vi "Block touchscreen.vi"(8 "error in (no error)":errorcluster, 10 "Block touchscreen?":bool, 11 "VISA resource name":refnum<visa-resource-name>) -> (0 "error out":errorcluster, 3 "VISA resource name out":refnum<visa-resource-name>)   [LabVIEW 2017, in "Sefram DAS220.lvlib"]
doc: "Lock or unlock the device touchscreen."
uses:
  <instrlib>/Sefram DAS220/Sefram DAS220.lvlib
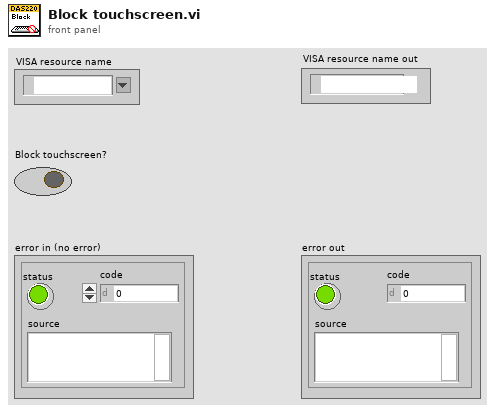
[diagram p1: front panel]
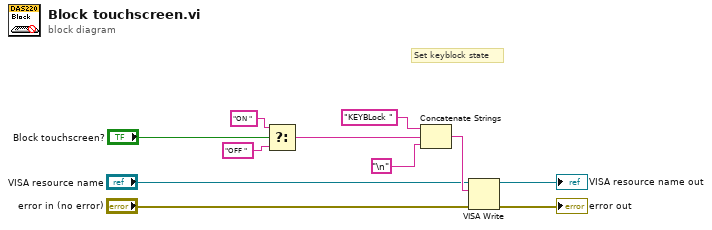
[diagram p0: block diagram]
diagram:
  # "Set keyblock state"
  n1 = Select(t="ON " ("string"), s="Block touchscreen?", f="OFF " ("string")) -> (s? t:f=w1:string)
  n2 = Concatenate Strings("KEYBLock " ("string"), w1, "\n") -> (w11:string)
  n3 = VISA Write(VISA resource name="VISA resource name", write buffer=w11, error in (no error)="error in (no error)") -> (VISA resource name out=→"VISA resource name out":refnum<visa-resource-name>, error out=→"error out":errorcluster)  [unwired: 1 out]
